vi "Create All Message Queues.vi"(8 "error in (no error)":errorcluster) -> (0 "error out":errorcluster, 3 "Message Queues out":T1)   [LabVIEW 2017, in "Front Panel Message Queue.lvlib"]
doc: "This VI creates and initializes all the message queues for your application. If your application requires more than one message queue, right-click the \"Message Queues\" constant above and select Open Type Def. Add the new Message Queue(s) to the type definition, then initialize them in this VI."
uses:
  Front Panel Message Queue.lvlib
  Example Message Queues.ctl
  Message Cluster.ctl
  Enqueue Message (Single).vi
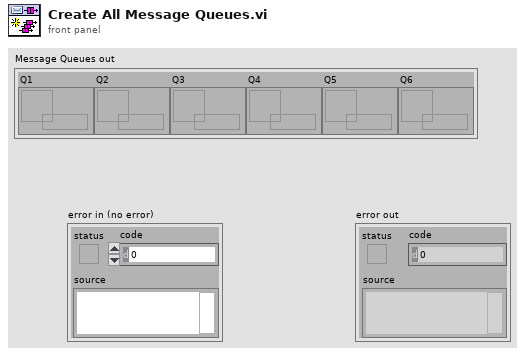
[diagram p1: front panel]
types:
  T1 = typedef "Front Panel Message Queue.lvlib/Example Message Queues.ctl" = cluster{"Q1":refnum<queue>, "Q2":refnum<queue>, "Q3":refnum<queue>, "Q4":refnum<queue>, "Q5":refnum<queue>, "Q6":refnum<queue>}
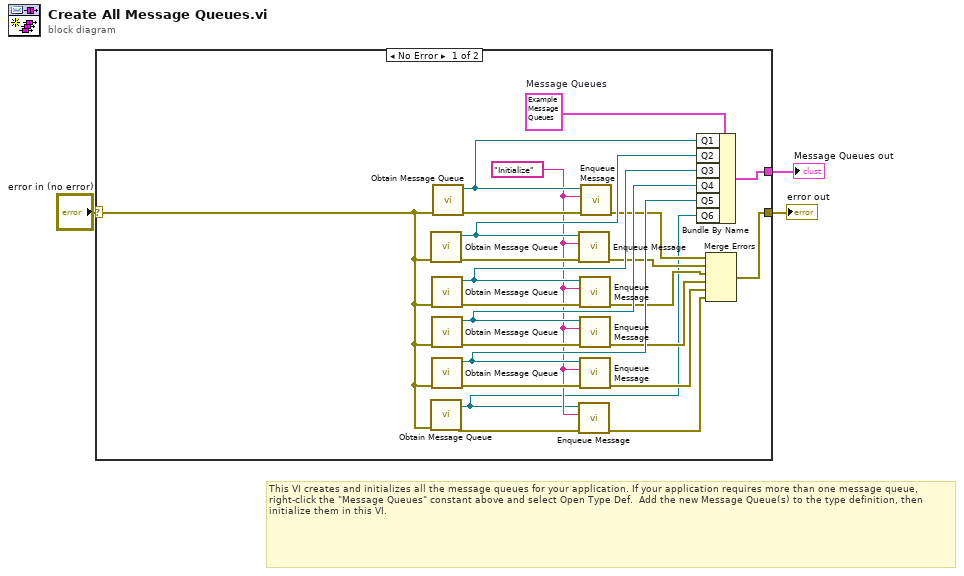
[diagram p0: block diagram]
diagram:
  # "This VI creates and initializes all the message queues for your application. If your application requires more than one message queue, right-click the \"Message Queues\" constant above and select Open Type Def.  Add the new Message Queue(s) to the type definition, then initialize them in this VI."
  n1 = case shown="No Error" "error in (no error)" {
    selector: "error in (no error)" -> [w6 w27]
    tunnel: [w14 w27] -> w3
    tunnel: [w25 _] -> w2
    frame No Error {
      w8 = "Initialize" ("Message")
      w26 = T1 {"Q1"=refnum, "Q2"=refnum, "Q3"=refnum, "Q4"=refnum, "Q5"=refnum, "Q6"=refnum}  # Message Queues
      n2 = call "Obtain Message Queue.vi"("error in (no error)"=w6) -> ("error out"=w22:errorcluster, "Message Queue"=w18:refnum<queue>)  [unwired: 9 in]
      n3 = call "Obtain Message Queue.vi"("error in (no error)"=w6) -> ("error out"=w7:errorcluster, "Message Queue"=w4:refnum<queue>)  [unwired: 9 in]
      n4 = call "Obtain Message Queue.vi"("error in (no error)"=w6) -> ("error out"=w21:errorcluster, "Message Queue"=w17:refnum<queue>)  [unwired: 9 in]
      n5 = call "Obtain Message Queue.vi"("error in (no error)"=w6) -> ("error out"=w20:errorcluster, "Message Queue"=w16:refnum<queue>)  [unwired: 9 in]
      n6 = call "Obtain Message Queue.vi"("error in (no error)"=w6) -> ("error out"=w19:errorcluster, "Message Queue"=w15:refnum<queue>)  [unwired: 9 in]
      n7 = call "Obtain Message Queue.vi"("error in (no error)"=w6) -> ("error out"=w24:errorcluster, "Message Queue"=w23:refnum<queue>)  [unwired: 9 in]
      n8 = call-poly "Enqueue Message.vi"("error in (no error)"=w22, "Message"=w8, "Message Queue"=w18) -> ("error out"=w12:errorcluster)  [unwired: 7 in, 1 out]
      n9 = call-poly "Enqueue Message.vi"("error in (no error)"=w7, "Message"=w8, "Message Queue"=w4) -> ("error out"=w5:errorcluster)  [unwired: 7 in, 1 out]
      n10 = call-poly "Enqueue Message.vi"("error in (no error)"=w21, "Message"=w8, "Message Queue"=w17) -> ("error out"=w11:errorcluster)  [unwired: 7 in, 1 out]
      n11 = call-poly "Enqueue Message.vi"("error in (no error)"=w20, "Message"=w8, "Message Queue"=w16) -> ("error out"=w10:errorcluster)  [unwired: 7 in, 1 out]
      n12 = call-poly "Enqueue Message.vi"("error in (no error)"=w19, "Message"=w8, "Message Queue"=w15) -> ("error out"=w9:errorcluster)  [unwired: 7 in, 1 out]
      n13 = call-poly "Enqueue Message.vi"("error in (no error)"=w24, "Message"=w8, "Message Queue"=w23) -> ("error out"=w13:errorcluster)  [unwired: 7 in, 1 out]
      n14 = Bundle By Name(cluster=w26, "Q1"=w23, "Q2"=w18, "Q3"=w17, "Q4"=w16, "Q5"=w15, "Q6"=w4) -> (w25:T1)
      n15 = Merge Errors(w13, w12, w11, w10, w9, w5) -> (w14:errorcluster)
    }
    frame Error {
    }
  }
  "Message Queues out" <- w2
  "error out" <- w3
